vi "WPI_UtilitiesFRC FPGAVersion.vi"(8 "error in (no error)":errorcluster) -> (0 "error out":errorcluster, 1 "Revision":u32, 2 "Version":u16=2009)   [LabVIEW 2017]
doc: "Returns the version and revision of the FPGA image on the CompactRIO device.\n\nThis software is licensed. Open the labview\\readme\\WPI Robotics Library Open Source License.txt file for more information."
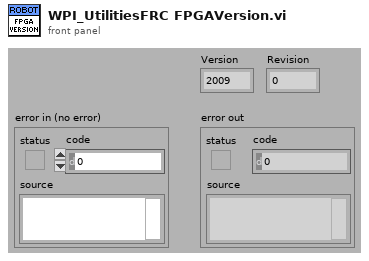
[diagram p1: front panel]
types:
  T1 = typedef "FPGA_GlobalDevRef.ctl" = cluster{"DevStatus":errorcluster}
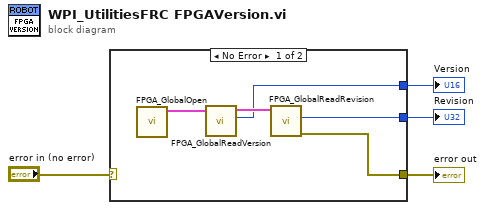
[diagram p0: block diagram]
diagram:
  n1 = case shown="No Error" "error in (no error)" {
    selector: "error in (no error)" -> [_ w10]
    tunnel: [w5 w10] -> w3
    tunnel: [w7 _] -> w2
    tunnel: [w6 _] -> w1
    frame No Error {
      n2 = call <vilib>:"FPGA_GlobalOpen.vi"() -> ("GlobalDevRef"=w9:T1)  [unwired: 2 in, 9 out]
      n3 = call <vilib>:"FPGA_GlobalReadVersion.vi"("GlobalDeviceRef In"=w9) -> ("Version"=w7:u16, "GlobalDeviceRef Out"=w8:T1)  [unwired: 1 in, 8 out]
      n4 = call <vilib>:"FPGA_GlobalReadRevision.vi"("GlobalDeviceRef In"=w8) -> ("error out"=w5:errorcluster, "Revision"=w6:u32)  [unwired: 1 in, 8 out]
    }
    frame Error {
    }
  }
  "error out" <- w3
  "Version" <- w2
  "Revision" <- w1
